vi "DataLoopback.vi"() -> ()   [LabVIEW 2011]
panel:
  out "data out":string
  in  "Port 2":u16=6342
  in  "Machine -Rx":string="localhost"
  out "Data Received":string
  in  "Port":u16=6341
  in  "Machine -Tx":string="localhost"
  in  "stop":bool
  in  "Send":bool
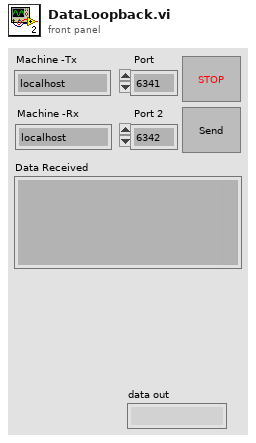
[diagram p1: front panel]
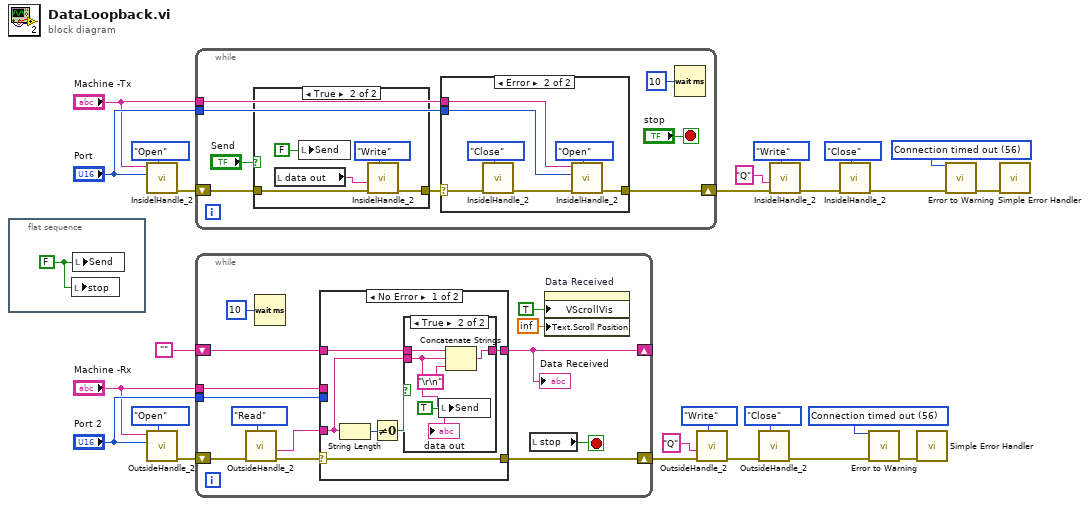
[diagram p0: block diagram]
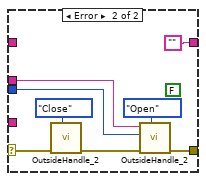
[diagram p3: hidden frame]
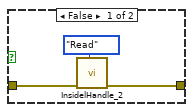
[diagram p4: hidden frame]
diagram:
  w11 = 56 items=["No Error", "Argument Error", "Memory Full", "Out of Zone", "End of File", "File Already Open", "Generic File IO Error", "File Not Found", "File Permission Error", "Disk Full", "Duplicate Path", "Too Many Files Open", "Not Enabled", "Resource File Not Found", "Cannot Add Resource", "Resource Not Found", "Image Not Found", "Image Memory Error", "Pen Does Not Exist", "Config Bad Type", "Config Token Not Found", "Config Parse Error", "Config Memory Error", "Bad External Code Format", "Bad External Code Offset", "External Code Not Present", "Null Window", "Destroy Window Mixup", "Null Menu", "Print Aborted", "Bad Print Record", "Print Driver Error", "Windows Error During Print", "Memory Error During Print", "Print Dialog Error", "Generic Print Error", "Invalid Device Refnum", "Device Not Found", "Device Parameter Error", "Device Unit Error", "Can't Open Device", "Device Call Aborted", "Generic Error", "Cancelled By User", "Object ID Too Low", "Object ID Too High", "Object Not In Heap", "Unknown Heap", "Bad DefProc ID", "DefProc Not In Table", "Message Out Of Range", "Null Method", "Unknown Message", "Manager Call Not Supported", "Bad address", "Connection In progress", "Connection timed out", "Connection is already in progress", "Network attribute not supported", "Network error", "Address in use", "System out of memory", "Connection aborted", "Connection refused", "Connection is not connected", "Connection is already connected", "Connection closed", "Initialize error (interapplication manager)", "Bad occurrence", "Wait on unbound occurrence handler", "Occurrence queue overflow", "Bad path", "Semaphore not signaled", "Unrecognized type (interapplication manager)"] ("1st Error to Convert")
  w23 = 56 items=["No Error", "Argument Error", "Memory Full", "Out of Zone", "End of File", "File Already Open", "Generic File IO Error", "File Not Found", "File Permission Error", "Disk Full", "Duplicate Path", "Too Many Files Open", "Not Enabled", "Resource File Not Found", "Cannot Add Resource", "Resource Not Found", "Image Not Found", "Image Memory Error", "Pen Does Not Exist", "Config Bad Type", "Config Token Not Found", "Config Parse Error", "Config Memory Error", "Bad External Code Format", "Bad External Code Offset", "External Code Not Present", "Null Window", "Destroy Window Mixup", "Null Menu", "Print Aborted", "Bad Print Record", "Print Driver Error", "Windows Error During Print", "Memory Error During Print", "Print Dialog Error", "Generic Print Error", "Invalid Device Refnum", "Device Not Found", "Device Parameter Error", "Device Unit Error", "Can't Open Device", "Device Call Aborted", "Generic Error", "Cancelled By User", "Object ID Too Low", "Object ID Too High", "Object Not In Heap", "Unknown Heap", "Bad DefProc ID", "DefProc Not In Table", "Message Out Of Range", "Null Method", "Unknown Message", "Manager Call Not Supported", "Bad address", "Connection In progress", "Connection timed out", "Connection is already in progress", "Network attribute not supported", "Network error", "Address in use", "System out of memory", "Connection aborted", "Connection refused", "Connection is not connected", "Connection is already connected", "Connection closed", "Initialize error (interapplication manager)", "Bad occurrence", "Wait on unbound occurrence handler", "Occurrence queue overflow", "Bad path", "Semaphore not signaled", "Unrecognized type (interapplication manager)"] ("1st Error to Convert")
  n1 = flat-sequence {
    frame #0 {
      w26 = FALSE ("Send")
      n2 = local write "stop"(w26) -> ()
      n3 = local write "Send"(w26) -> ()
    }
  }
  n4 = call "InsidelHandle_2.vi"("Mode"=enum16{"Open", "Read", "Write", "Close"}."Open", "Port"="Port", "Machine"="Machine -Tx") -> ("error out"=w15:errorcluster)  [unwired: 7 in, 1 out]
  n5 = call "OutsideHandle_2.vi"("Mode"=enum16{"Open", "Read", "Write", "Close"}."Open", "Port"="Port 2", "Machine"="Machine -Rx") -> ("error out"=w2:errorcluster)  [unwired: 7 in, 1 out]
  n6 = while {
    shift-right: [w33] -> w19
    shift-left: w15 -> [w32]
    tunnel: "Machine -Tx" -> [w30]
    tunnel: "Port" -> [w29]
    stop <- "stop" stop-if-true
    n7 = case shown="True" "Send" {
      tunnel: w32 -> [w36 w42]
      tunnel: [w35 w41] -> w31
      frame False {
        n8 = call "InsidelHandle_2.vi"("Mode"=enum16{"Open", "Read", "Write", "Close"}."Read", "error in (no error)"=w36) -> ("error out"=w35:errorcluster)  [unwired: 8 in, 1 out]
      }
      frame True {
        n9 = local read "data out"() -> (w38:string)
        n10 = local write "Send"(FALSE ("Send")) -> ()
        n11 = call "InsidelHandle_2.vi"("Mode"=enum16{"Open", "Read", "Write", "Close"}."Write", "error in (no error)"=w42, "data in"=w38) -> ("error out"=w41:errorcluster)  [unwired: 7 in, 1 out]
      }
    }
    n12 = case shown="Error" w31 {
      selector: w31 -> [w43 w46]
      tunnel: [w43 w47] -> w33
      tunnel: w30 -> [_ w45]
      tunnel: w29 -> [_ w44]
      frame No Error {
      }
      frame Error {
        n13 = call "InsidelHandle_2.vi"("Mode"=enum16{"Open", "Read", "Write", "Close"}."Close", "error in (no error)"=w46) -> ("error out"=w48:errorcluster)  [unwired: 8 in, 1 out]
        n14 = call "InsidelHandle_2.vi"("Mode"=enum16{"Open", "Read", "Write", "Close"}."Open", "error in (no error)"=w48, "Port"=w44, "Machine"=w45) -> ("error out"=w47:errorcluster)  [unwired: 6 in, 1 out]
      }
    }
    n15 = Wait (ms)(milliseconds to wait=u32 10) -> ()  [unwired: 1 out]
  }
  n16 = while {
    shift-right: [w62] -> w6
    shift-left: w2 -> [w60]
    shift-right: [w54] -> _
    shift-left: "" -> [w61]
    tunnel: "Machine -Rx" -> [w56]
    tunnel: "Port 2" -> [w55]
    stop <- w51 stop-if-true
    n17 = call "OutsideHandle_2.vi"("Mode"=enum16{"Open", "Read", "Write", "Close"}."Read", "error in (no error)"=w60) -> ("error out"=w59:errorcluster, "data out"=w58:string)  [unwired: 8 in]
    n18 = Wait (ms)(milliseconds to wait=u32 10) -> ()  [unwired: 1 out]
    n19 = case shown="No Error" w59 {
      selector: w59 -> [w69 w79]
      tunnel: [w69 w80] -> w62
      tunnel: w58 -> [w65 _]
      tunnel: w61 -> [w66 _]
      tunnel: [w64 ""] -> w54
      tunnel: w56 -> [_ w77]
      tunnel: w55 -> [_ w76]
      frame No Error {
        n20 = String Length(string=w65) -> (length=w68:i32)
        n21 = Not Equal To 0?(x=w68) -> (x != 0?=w67:bool)
        n22 = case shown="True" w67 {
          tunnel: w66 -> [w70 w75]
          tunnel: w65 -> [_ w71]
          tunnel: [w70 w74] -> w64
          frame False {
          }
          frame True {
            n23 = local write "Send"(TRUE ("Send")) -> ()
            n24 = Concatenate Strings(w75, w71, "\r\n" ("Substring")) -> (w74:string)
            "data out" <- w71
          }
        }
      }
      frame Error {
        (unwired) FALSE ("Send")
        n25 = call "OutsideHandle_2.vi"("Mode"=enum16{"Open", "Read", "Write", "Close"}."Close", "error in (no error)"=w79) -> ("error out"=w81:errorcluster)  [unwired: 8 in, 1 out]
        n26 = call "OutsideHandle_2.vi"("Mode"=enum16{"Open", "Read", "Write", "Close"}."Open", "error in (no error)"=w81, "Port"=w76, "Machine"=w77) -> ("error out"=w80:errorcluster)  [unwired: 6 in, 1 out]
      }
    }
    "Data Received" <- w54
    n27 = local read "stop"() -> (w51:bool)
    n28 = property on="Data Received" class="Str"("VScrollVis"=TRUE ("Vertical Scrollbar Visible"), "Text.Scroll Position"=inf) -> ()  [unwired: 2 in, 2 out]
  }
  n29 = call "OutsideHandle_2.vi"("Mode"=enum16{"Open", "Read", "Write", "Close"}."Write", "error in (no error)"=w6, "data in"="Q") -> ("error out"=w5:errorcluster)  [unwired: 7 in, 1 out]
  n30 = call "OutsideHandle_2.vi"("Mode"=enum16{"Open", "Read", "Write", "Close"}."Close", "error in (no error)"=w5) -> ("error out"=w12:errorcluster)  [unwired: 8 in, 1 out]
  n31 = call "InsidelHandle_2.vi"("Mode"=enum16{"Open", "Read", "Write", "Close"}."Write", "error in (no error)"=w19, "data in"="Q") -> ("error out"=w18:errorcluster)  [unwired: 7 in, 1 out]
  n32 = call "InsidelHandle_2.vi"("Mode"=enum16{"Open", "Read", "Write", "Close"}."Close", "error in (no error)"=w18) -> ("error out"=w24:errorcluster)  [unwired: 8 in, 1 out]
  n33 = call <vilib>:"Error to Warning.vi"("1st Error to Convert"=w11, "error in"=w12) -> ("warning out"=w13:errorcluster)  [unwired: 3 in, 10 out]
  n34 = call <vilib>:"Simple Error Handler.vi"("error in (no error)"=w13) -> ()  [unwired: 1 in, 8 out]
  n35 = call <vilib>:"Error to Warning.vi"("1st Error to Convert"=w23, "error in"=w24) -> ("warning out"=w25:errorcluster)  [unwired: 3 in, 10 out]
  n36 = call <vilib>:"Simple Error Handler.vi"("error in (no error)"=w25) -> ()  [unwired: 1 in, 8 out]
